vi "Variablen-Textanzeige.vi"(9 "Param Ziffernanzeige":T1={"Wert-String"="123,4567", "Rechteck"={"left"=10, "top"=10, "right"=90, "bottom"=30}, "Schriftgröße"=18, "Textfarbe"=16776769, "Hintergrund"=16730368, "Rahmenfarbe"=16730368}, 11 "Bild":picture caption="Grafik") -> (3 "Bild neu":picture)   [LabVIEW 2020, in "Anlagenuebersicht.lvlib" / "VisBx Anzeige.lvlib"]
uses:
  VisBx Anzeige.lvlib
  VisParameter/Param Ziffernanzeige.ctl
  VisParameter/VisParam-Typdef.lvlib
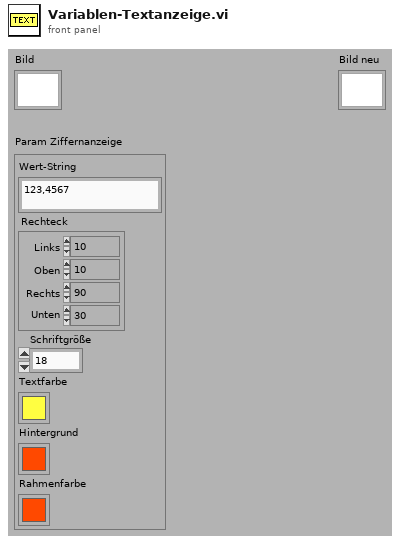
[diagram p1: front panel]
types:
  T1 = typedef "VisParam-Typdef.lvlib/Param Ziffernanzeige.ctl" = cluster{"Wert-String":string, "Rechteck":cluster{"left":i16, "top":i16, "right":i16, "bottom":i16}, "Schriftgröße":i16, "Textfarbe":u32, "Hintergrund":u32, "Rahmenfarbe":u32}
  T2 = cluster{"left":i16, "top":i16, "right":i16, "bottom":i16}
  T3 = cluster{"Font Name:":string, "Size":i16, "Strikeout?":bool, "Italic?":bool, "Underline?":bool, "Outline?":bool, "Shadow?":bool, "Bold?":bool}
  T4 = enum16{"User-specified Font", "Application Font", "System Font", "Dialog Font"}
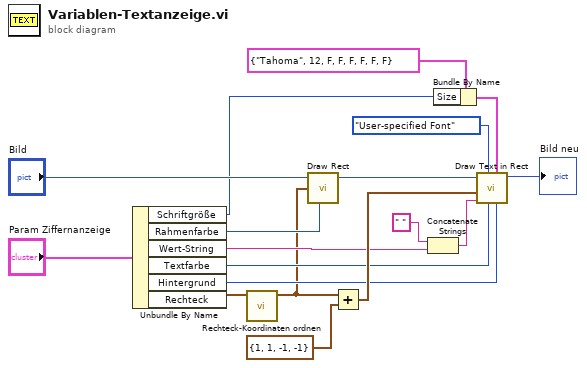
[diagram p0: block diagram]
diagram:
  n1 = Unbundle By Name("Param Ziffernanzeige") -> ("Schriftgröße"=w9:i16, "Rahmenfarbe"=w6:u32, "Wert-String"=w4:string, "Textfarbe"=w8:u32, "Hintergrund"=w7:u32, "Rechteck"=w2:T2)
  n2 = call "Rechteck-Koordinaten ordnen.vi"("Rechteck-Koordinaten"=w2) -> ("Koordinaten geordnet"=w1:T2)  [unwired: 6 in]
  n3 = call <vilib>:"Draw Rect.vi"("picture"="Bild", "rect"=w1, "color(black)"=w6) -> ("new picture"=w14:picture)  [unwired: 2 in, 4 out]
  n4 = Add(x=w1, y=T2 {"left"=1, "top"=1, "right"=-1, "bottom"=-1} ("Rechteck")) -> (x+y=w13:T2)
  n5 = Concatenate Strings(" ", w4) -> (w3:string)
  n6 = Bundle By Name(cluster=T3 {"Font Name:"="Tahoma", "Size"=12, "Strikeout?"=FALSE, "Italic?"=FALSE, "Underline?"=FALSE, "Outline?"=FALSE, "Shadow?"=FALSE, "Bold?"=FALSE} ("[user-specified font]"), "Size"=w9) -> (w16:T3)
  n7 = call <vilib>:"Draw Text in Rect.vi"("BG color(transparent)"=w7, "[user-specified font]"=w16, "text color(black)"=w8, "desired font(Application)"=T4."User-specified Font", "text"=w3, "rect"=w13, "picture"=w14) -> ("new picture"=→"Bild neu":picture)  [unwired: 1 in, 3 out]
